vi "MARS3D Experiment Time.vi"(8 "Time Experiment":string, 11 "Time Calibration":string) -> (2 "Time elapsed (MIN)":dbl)   [LabVIEW 2013]
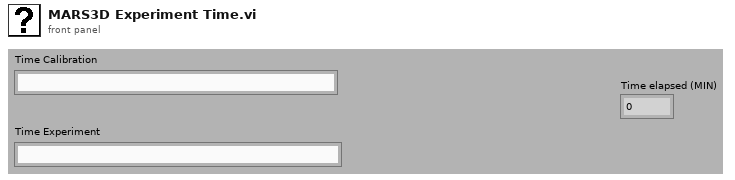
[diagram p1: front panel]
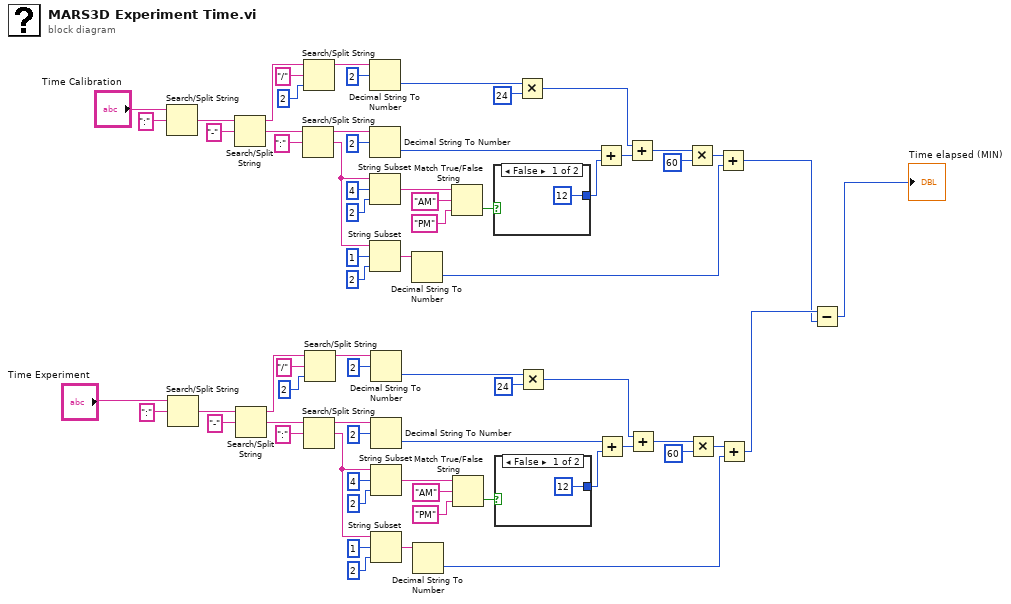
[diagram p0: block diagram]
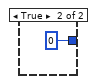
[diagram p2: hidden frame]
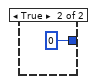
[diagram p3: hidden frame]
diagram:
  n1 = Search/Split String(string="Time Calibration", search string/char (-)=":") -> (match + rest of string=w66:string)  [unwired: 1 in, 2 out]
  n2 = Search/Split String(string="Time Experiment", search string/char (-)=":") -> (match + rest of string=w34:string)  [unwired: 1 in, 2 out]
  n3 = Search/Split String(string=w66, search string/char (-)="-") -> (substring before match=w46:string, match + rest of string=w64:string)  [unwired: 1 in, 1 out]
  n4 = Search/Split String(string=w34, search string/char (-)="-") -> (substring before match=w14:string, match + rest of string=w32:string)  [unwired: 1 in, 1 out]
  n5 = Search/Split String(string=w64, search string/char (-)=":") -> (substring before match=w62:string, match + rest of string=w53:string)  [unwired: 1 in, 1 out]
  n6 = Search/Split String(string=w46, search string/char (-)="/", offset (0)=2) -> (substring before match=w43:string)  [unwired: 2 out]
  n7 = Search/Split String(string=w32, search string/char (-)=":") -> (substring before match=w30:string, match + rest of string=w21:string)  [unwired: 1 in, 1 out]
  n8 = Search/Split String(string=w14, search string/char (-)="/", offset (0)=2) -> (substring before match=w11:string)  [unwired: 2 out]
  n9 = Decimal String To Number(string=w43, offset=2) -> (number=w41:i32)  [unwired: 1 in, 1 out]
  n10 = Decimal String To Number(string=w62, offset=2) -> (number=w47:i32)  [unwired: 1 in, 1 out]
  n11 = String Subset(string=w53, offset (0)=4, length (rest)=2 ("length (rest)")) -> (substring=w52:string)
  n12 = String Subset(string=w53, offset (0)=1, length (rest)=2 ("length (rest)")) -> (substring=w56:string)
  n13 = Decimal String To Number(string=w11, offset=2) -> (number=w9:i32)  [unwired: 1 in, 1 out]
  n14 = Decimal String To Number(string=w30, offset=2) -> (number=w15:i32)  [unwired: 1 in, 1 out]
  n15 = String Subset(string=w21, offset (0)=4, length (rest)=2 ("length (rest)")) -> (substring=w20:string)
  n16 = String Subset(string=w21, offset (0)=1, length (rest)=2 ("length (rest)")) -> (substring=w24:string)
  n17 = Decimal String To Number(string=w56) -> (number=w59:i32)  [unwired: 2 in, 1 out]
  n18 = Decimal String To Number(string=w24) -> (number=w27:i32)  [unwired: 2 in, 1 out]
  n19 = Match True/False String(2:"PM" ("false string"), 3:"AM" ("true string"), 4:w52) -> (0:w49:bool)  [unwired: 1 out]
  n20 = Match True/False String(2:"PM" ("false string"), 3:"AM" ("true string"), 4:w20) -> (0:w17:bool)  [unwired: 1 out]
  n21 = case shown="False" w49 {
    tunnel: [12 0] -> w48
    frame False {
    }
    frame True {
    }
  }
  n22 = case shown="False" w17 {
    tunnel: [12 0] -> w16
    frame False {
    }
    frame True {
    }
  }
  n23 = Multiply(x=w41, y=24) -> (x*y=w39:i32)
  n24 = Multiply(x=w9, y=24) -> (x*y=w7:i32)
  n25 = Add(x=w47, y=w48) -> (x+y=w42:i32)
  n26 = Add(x=w15, y=w16) -> (x+y=w10:i32)
  n27 = Add(x=w39, y=w42) -> (x+y=w38:i32)
  n28 = Add(x=w7, y=w10) -> (x+y=w6:i32)
  n29 = Multiply(x=w38, y=60) -> (x*y=w60:i32)
  n30 = Multiply(x=w6, y=60) -> (x*y=w28:i32)
  n31 = Add(x=w60, y=w59) -> (x+y=w2:i32)
  n32 = Add(x=w28, y=w27) -> (x+y=w3:i32)
  n33 = Subtract(x=w3, y=w2) -> (x-y=→"Time elapsed (MIN)":i32)
